vi "1.Main demo.vi"() -> ()   [LabVIEW 2013]
uses:
  UnderAutomation.Fanuc/UnderAutomation.Fanuc.lvlib
  C:/Users/fg/Documents/Fanuc.vi/LabVIEW_2024/UnderAutomation.Fanuc/lib/UnderAutomation.Fanuc.dll
  LabVIEW_2024/UnderAutomation.Fanuc/lib/UnderAutomation.Fanuc.dll
panel:
  out "SNPX connected":bool
  out "FTP connected":bool
  out "Telnet connected":bool
  in  "Tab Control":T1(tab)
  in  "Disconnect":bool
  in  "Test":bool
  in  "Key":string
  in  "Licensee":string
  in  "Use SNPX":bool
  in  "FTP password":string
  in  "FTP user":string
  in  "Use FTP":bool
  in  "Connect":bool
  in  "Telnet password":string
  in  "Use Telnet":bool
  in  "ConnectRoboguide":bool
  in  "RoboguideRobotPath":path caption="Path to \"Robot\" ROBOGUIDE folder that contains services.txt"
  in  "IP":string caption="Robot IP Address"
  out "License state":string
  out "Connect error":string
  in  "Unsimulate all":bool
  in  "Unsimulate":bool
  in  "Simulate":bool
  in  "Set port value":bool
  in  "Variable set value":bool
  in  "Variable new value":string caption="New value"
  in  "Variable get value":bool
  in  "Variable name":string
  out "Telnet warning":string
  out "Current position":T2
  in  "Get current position":bool
  in  "Reset alarms":bool
  in  "Get task info":bool
  in  "Task name":string caption="Task name (program without extension)"
  in  "Abort all programs":bool
  in  "Clear variable":bool
  in  "Clear Program":bool
  in  "Hold":bool
  in  "Continue":bool
  in  "Abort":bool
  in  "Pause":bool
  in  "Program name":string caption="Program name without extension"
  in  "Run":bool
  out "TelnetError":string caption="Error :"
  out "TelnetSucceed":bool caption="Succeeded"
  out "KclCommand":string caption="Last command :"
  out "TaskInfo":T3
  out "Variable value":string
  in  "port":i32(ring) items=["DIN", "DOUT", "RDO", "OPOUT", "TPOUT", "WDI", "WDO", "AIN", "AOUT", "GIN", "GOUT"]
  in  "index":i32
  in  "value":i32
  out "FTP warning":string
  out "PosReg":T4(array[cluster])
  out "StrReg":string[](array[string])
  in  "Tab Control IO state":T5(tab)
  out "UI":cluster{"Id":i32, "Name":string, "Value":bool}[](array[cluster])
  out "UO":cluster{"Id":i32, "Name":string, "Value":bool}[](array[cluster])
  out "SI":cluster{"Id":i32, "Name":string, "Value":bool}[](array[cluster])
  out "SO":cluster{"Id":i32, "Name":string, "Value":bool}[](array[cluster])
  out "DIN":cluster{"Id":i32, "Name":string, "Value":bool}[](array[cluster])
  out "DOUT":cluster{"Id":i32, "Name":string, "Value":bool}[](array[cluster])
  out "RI":cluster{"Id":i32, "Name":string, "Value":bool}[](array[cluster])
  out "RO":cluster{"Id":i32, "Name":string, "Value":bool}[](array[cluster])
  out "FLG":cluster{"Id":i32, "Name":string, "Value":bool}[](array[cluster])
  in  "Tab Control position":enum32{"World", "Joints", "User frames"}(tab)
  out "World Positions":T6(array[cluster])
  out "JointsPosition":dbl[](array[numeric])
  out "UserFramePositions":T7(array[cluster])
  in  "Get current position":bool
  in  "Get IO State":bool
  in  "Port":i32(ring) items=["DIN", "DOUT", "UI", "UO", "SI", "SO", "RI", "RO", "FLG"]
  out "Errors":T8(array[cluster])
  in  "Get all errors":bool
  in  "Get safety status":bool
  out "SafetyStatus":T9
  out "NumReg":dbl[](array[numeric])
  in  "Get numeric registers":bool
  in  "Get string registers":bool
  in  "Get position registers":bool
  out "SNPX warning":string
  in  "Tab Control snpx register":enum32{"Cartesian", "Joints"}(tab)
  in  "Cartesian position 2":T10
  in  "Write cartesian position register":bool
  in  "Joints position":dbl[](array[numeric])
  in  "Write joints position register":bool
  in  "Position register":i32
  in  "Read position register":bool
  out "Value":string
  in  "New value":string
  in  "String register":i32
  in  "Read string register":bool
  in  "Write string register":bool
  in  "Continuous read world position":bool
  out "JointsPosition":dbl[](array[numeric])
  out "Cartesian position":T11
  out "UserTool":i16
  out "error out":errorcluster
  in  "Continuous read user frame position":bool
  in  "userFrame":i32
  out "Cartesian position":T11
  out "UserTool":i16
  out "error out 2":errorcluster
  in  "Numeric register":i32
  in  "New value":sgl
  out "Value":sgl
  in  "Read numeric register":bool
  in  "Write numeric register":bool
  out "UserFrame":i16
  out "UserTool":i16
  in  "stop":bool
  out "Snpx":refnum<k24>
  out "Ftp":refnum<k24>
  out "Telnet":refnum<k24>
  out "robot":refnum<k24>
  # "UnderAutomation"
  # "https://underautomation.com/fanuc"
  # "+"
  # "LabVIEW demo app for remote control and monitoring of your Fanuc robot"
  # "Connect to robot"
  # "2. Ensure you have a trial or lifetime valid license"
  # "1. Set Fanuc robot address"
  # "This is a commercial library, you have a 30-day trial period. But you can use it forever if you buy a perpetual licence for your company (regardless of the number of robot, applications or developers)."
  # "Connect to real robot"
  # "Connect to ROBOGUIDE"
  # "If you have a license :"
  # "3. Select the services you want to connect to"
  # "Telnet"
  # "FTP"
  # "SNPX"
  # "You need option R553 \"HMI Device SNPX\" or R651 FRL"
  # "How to enable Telnet : https://underautomation.com/fanuc/documentation/enable-telnet"
  # "See : https://underautomation.com/fanuc/documentation/snpx"
  # "4. Connect to the robot"
  # "Telnet"
  # "Variables"
  # "Program execution"
  # "Task"
  # "Ports"
  # "Current position"
  # "Alarms"
  # "FTP"
  # "Current Position"
  # "IO State"
  # "Errors"
  # "Registers"
  # "Safety status"
  # "SNPX"
  # "Numeric registers"
  # "String registers"
  # "Read world position"
  # "Read user frame position"
  # "Position registers"
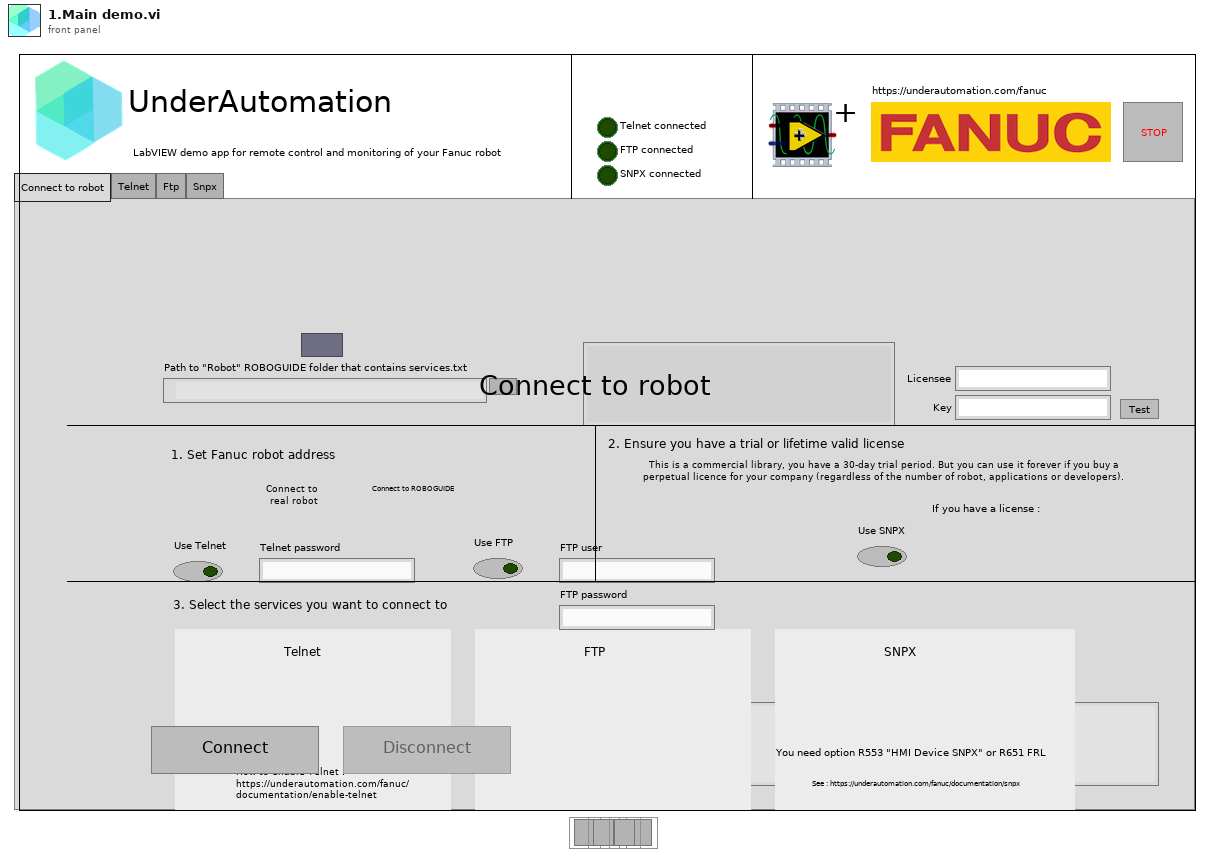
[diagram p1: front panel]
types:
  T1 = enum32{"Connect to robot", "Telnet", "Ftp", "Snpx"}
  T2 = cluster{"X":dbl, "Y":dbl, "Z":dbl, "W":dbl, "P":dbl, "R":dbl}
  T3 = cluster{"CurrentLine":i32, "RoutineName":string, "SystemTask":bool, "TaskName":string, "TaskNumber":i32, "TaskStatus":i32, "TaskStatusStr":string}
  T4 = cluster{"X":dbl, "Y":dbl, "Z":dbl, "W":dbl, "R":dbl, "P":dbl}[][]
  T5 = enum32{"UI", "UO", "SI", "SO", "DIN", "DOUT", "RI", "RO", "FLG"}
  T6 = cluster{"Tool":i32, "Cartesian position":cluster{cluster{"ArmFrontBack":i32, "ArmLeftRight":i32, "ArmUpDown":i32, "TurnAxis1":i32, "TurnAxis2":i32, "TurnAxis3":i32, "WristFlip":i32}, "X":dbl, "Y":dbl, "Z":dbl, "W":dbl, "P":dbl, "R":dbl}}[]
  T7 = cluster{"Frame":i32, "Tool":i32, "Cartesian position":cluster{cluster{"ArmFrontBack":i32, "ArmLeftRight":i32, "ArmUpDown":i32, "TurnAxis1":i32, "TurnAxis2":i32, "TurnAxis3":i32, "WristFlip":i32}, "X":dbl, "Y":dbl, "Z":dbl, "W":dbl, "P":dbl, "R":dbl}}[]
  T8 = cluster{"Id":i32, "IsReset":bool, "Text":string}[]
  T9 = cluster{"BeltBroken":bool, "ExternalEStop":bool, "FenceOpen":bool, "HandBroken":bool, "LowAirAlarm":bool, "NonTeacherEnb":bool, "OverTravel":bool, "SOPEStop":bool, "SVOFFDetect":bool, "TPDeadman":bool, "TPEnable":bool, "TPEStop":bool}
  T10 = cluster{"Configuration":cluster{"ArmFrontBack":i32, "ArmLeftRight":i32, "ArmUpDown":i32, "TurnAxis1":i32, "TurnAxis2":i32, "TurnAxis3":i32, "WristFlip":i32}, "X":dbl, "Y":dbl, "Z":dbl, "W":dbl, "P":dbl, "R":dbl}
  T11 = cluster{"Cartesian position":cluster{cluster{"ArmFrontBack":i32, "ArmLeftRight":i32, "ArmUpDown":i32, "TurnAxis1":i32, "TurnAxis2":i32, "TurnAxis3":i32, "WristFlip":i32}, "X":dbl, "Y":dbl, "Z":dbl, "W":dbl, "P":dbl, "R":dbl}, "Extension":cluster{"E1":dbl, "E2":dbl, "E3":dbl, "T4":i16, "T5":i16, "T6":i16}}
  T12 = enum8{"Enabled", "Disabled", "Disabled and Grayed Out"}
  T13 = cluster{"X":dbl, "Y":dbl, "Z":dbl, "W":dbl, "P":dbl, "R":dbl}[][]
  T14 = cluster{"Id":i32, "Values":dbl[], "UserFramePositions":cluster{"Frame":i32, "Tool":i32, "Cartesian position":cluster{cluster{"ArmFrontBack":i32, "ArmLeftRight":i32, "ArmUpDown":i32, "TurnAxis1":i32, "TurnAxis2":i32, "TurnAxis3":i32, "WristFlip":i32}, "X":dbl, "Y":dbl, "Z":dbl, "W":dbl, "P":dbl, "R":dbl}}[], "World Positions":cluster{"Tool":i32, "Cartesian position":cluster{cluster{"ArmFrontBack":i32, "ArmLeftRight":i32, "ArmUpDown":i32, "TurnAxis1":i32, "TurnAxis2":i32, "TurnAxis3":i32, "WristFlip":i32}, "X":dbl, "Y":dbl, "Z":dbl, "W":dbl, "P":dbl, "R":dbl}}[]}[]
  T15 = cluster{"Id":i32, "Name":string, "Port":i32, "Value":bool, "PortStr":string}[]
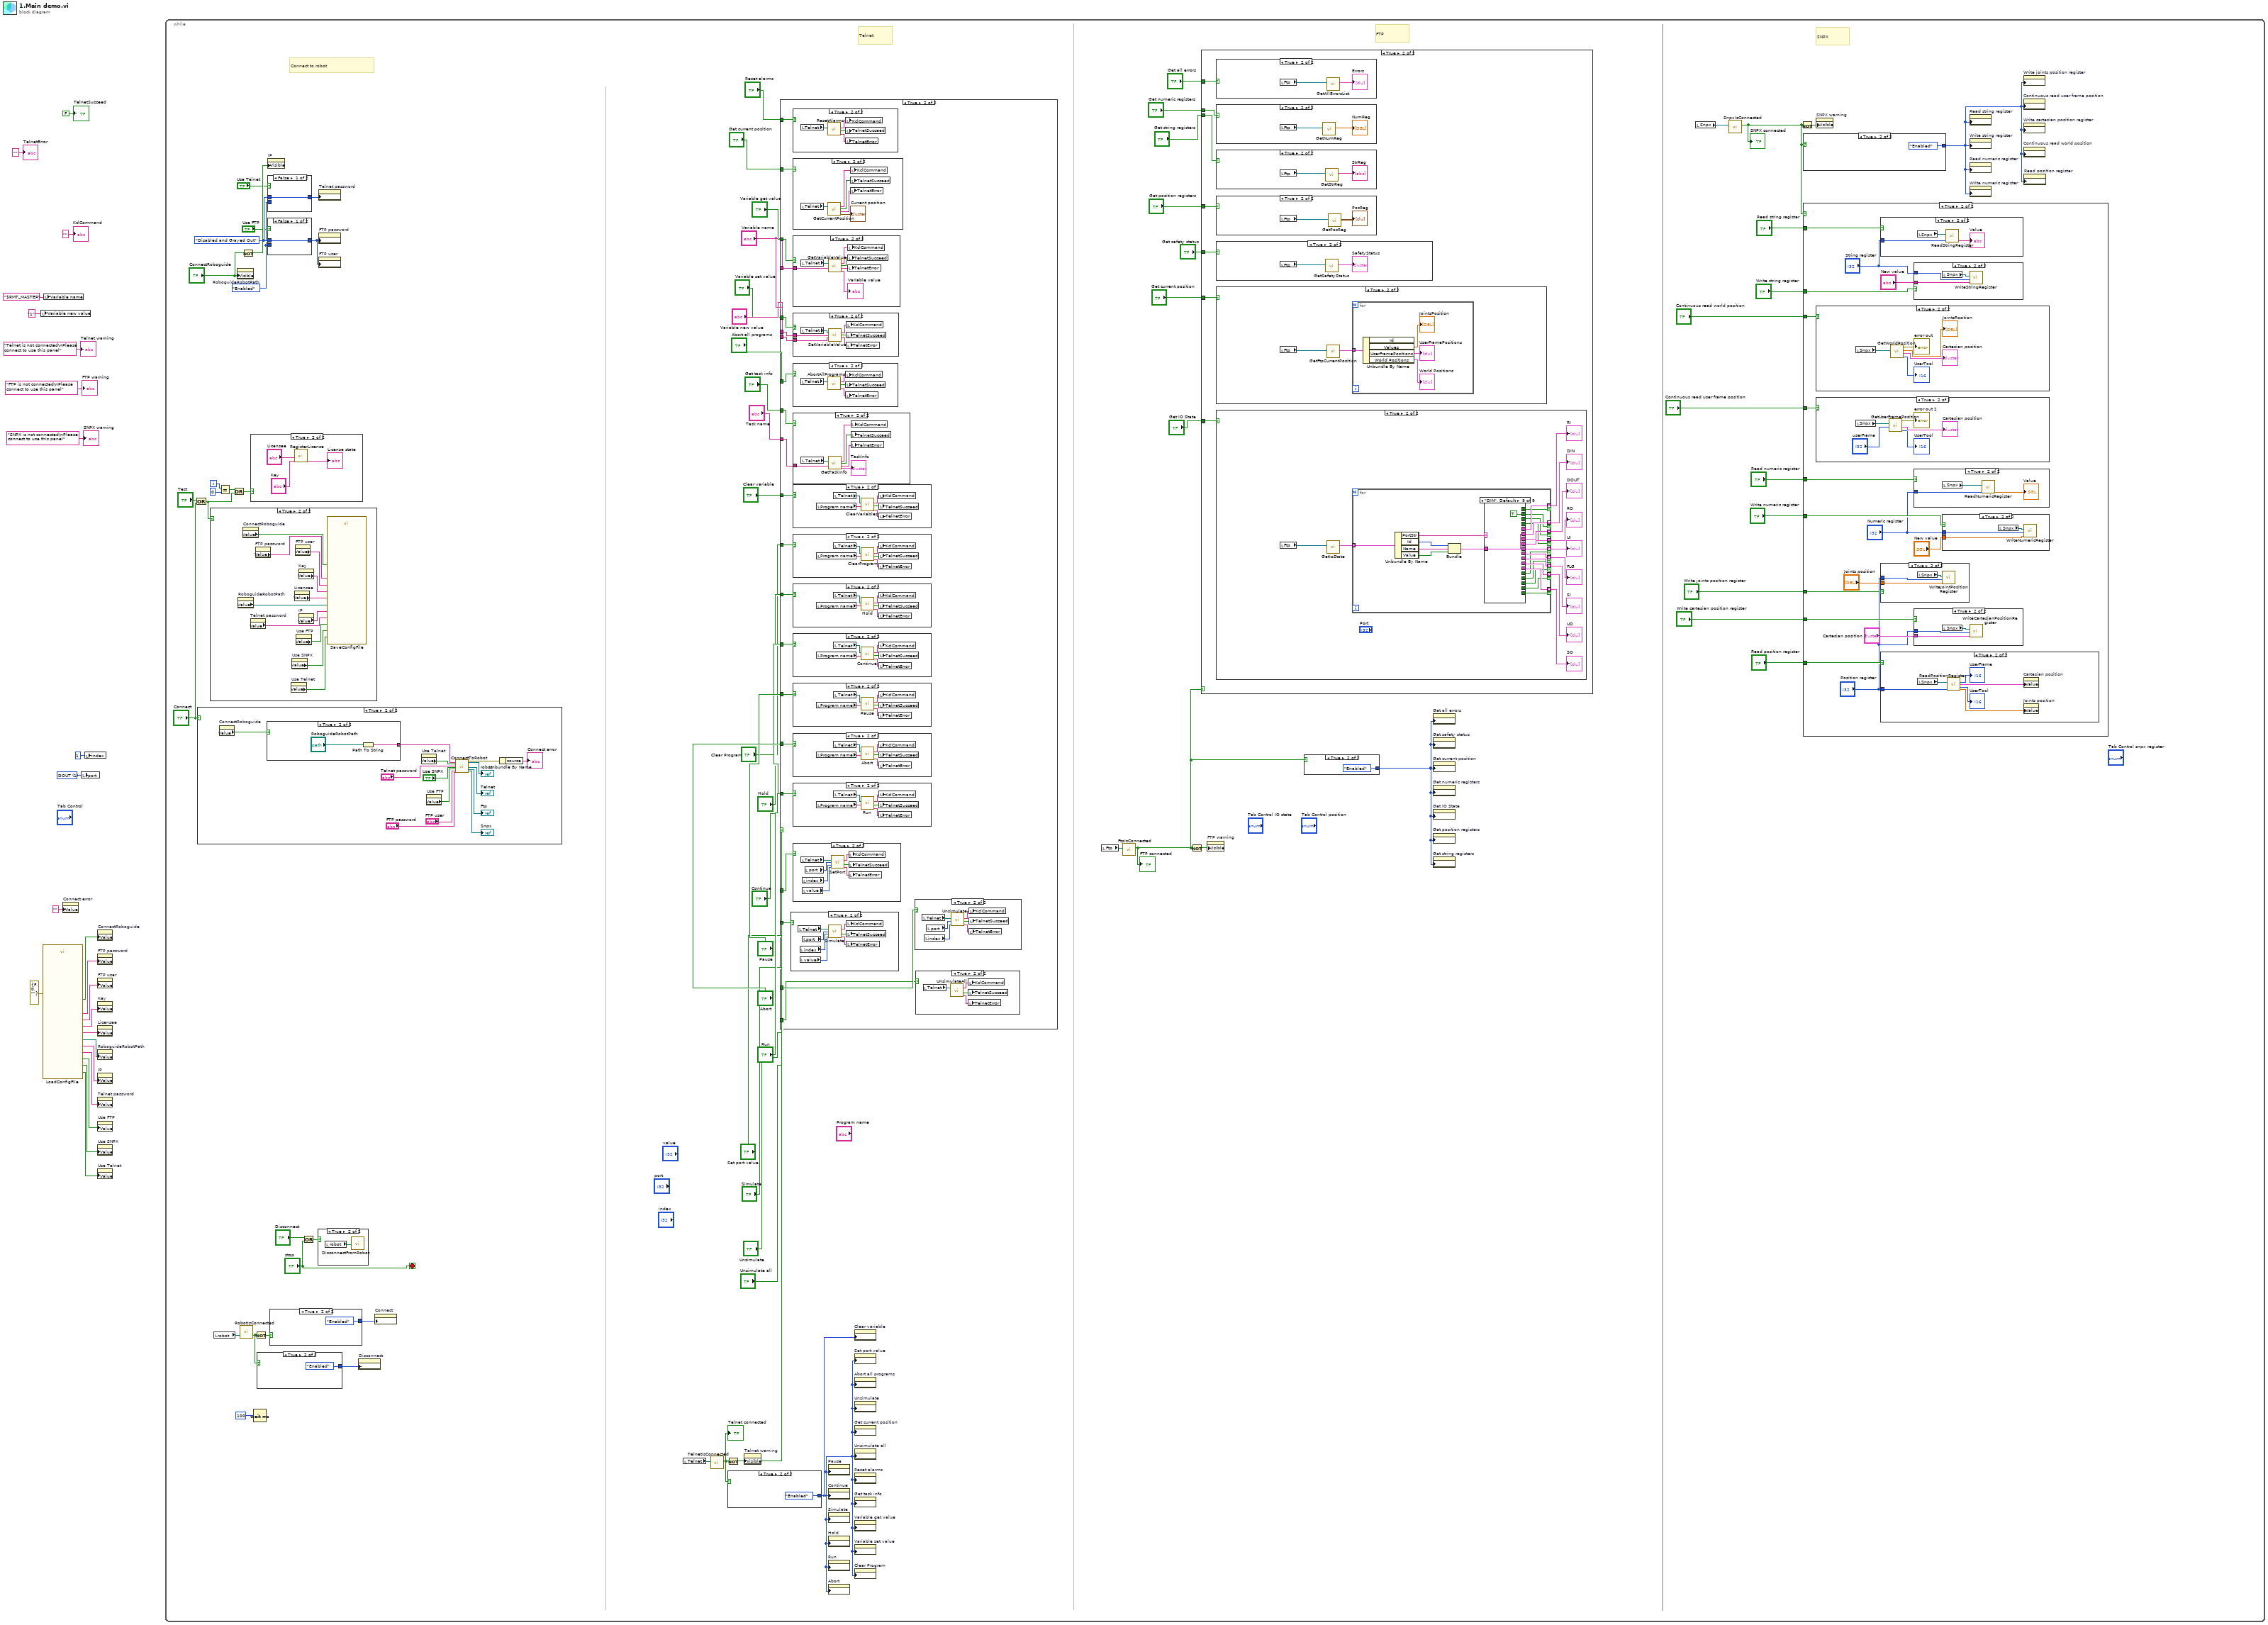
[diagram p0: block diagram]
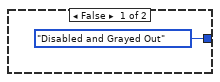
[diagram p2: hidden frame]
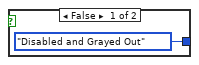
[diagram p13: hidden frame]
diagram:
  w3 = 1 items=["DIN", "DOUT", "RDO", "OPOUT", "TPOUT", "WDI", "WDO", "AIN", "AOUT", "GIN", "GOUT"] ("port")
  n1 = local write "Variable new value"("1" ("Variable new value")) -> ()
  n2 = call "LoadConfigFile.vi"("error in (no error)"=errorcluster {"status"=FALSE, "code"=0, "source"=""}) -> ("FTP password"=w20:string, "Licensee"=w12:string, "FTP user"=w19:string, "Key"=w13:string, "Use FTP"=w16:bool, "IP"=w22:string, "RoboguideRobotPath"=w18:path, "ConnectRoboguide"=w21:bool, "Use Telnet"=w14:bool, "Telnet password"=w17:string, "Use SNPX"=w15:bool)  [unwired: 15 in, 1 out]
  n3 = local write "Variable name"("$RMT_MASTER" ("Variable name")) -> ()
  n4 = property on="Connect error" class="Str"("Value"="" ("Connect error")) -> ()  [unwired: 2 in, 2 out]
  n5 = local write "port"(w3) -> ()
  n6 = local write "index"(1 ("index")) -> ()
  n7 = property on="ConnectRoboguide" class="Bool (strict)"("Value"=w21) -> ()  [unwired: 2 in, 2 out]
  n8 = property on="FTP password" class="Str"("Value"=w20) -> ()  [unwired: 2 in, 2 out]
  n9 = property on="FTP user" class="Str"("Value"=w19) -> ()  [unwired: 2 in, 2 out]
  n10 = property on="Key" class="Str"("Value"=w13) -> ()  [unwired: 2 in, 2 out]
  n11 = property on="Licensee" class="Str"("Value"=w12) -> ()  [unwired: 2 in, 2 out]
  n12 = property on="RoboguideRobotPath" class="Path"("Value"=w18) -> ()  [unwired: 2 in, 2 out]
  n13 = property on="IP" class="Str"("Value"=w22) -> ()  [unwired: 2 in, 2 out]
  n14 = property on="Telnet password" class="Str"("Value"=w17) -> ()  [unwired: 2 in, 2 out]
  n15 = property on="Use FTP" class="Bool (strict)"("Value"=w16) -> ()  [unwired: 2 in, 2 out]
  n16 = property on="Use SNPX" class="Bool (strict)"("Value"=w15) -> ()  [unwired: 2 in, 2 out]
  n17 = property on="Use Telnet" class="Bool (strict)"("Value"=w14) -> ()  [unwired: 2 in, 2 out]
  n18 = while {
    i -> [w90]
    stop <- "stop" stop-if-true
    w82 = T12."Enabled" ("Disabled")
    w83 = T12."Disabled and Grayed Out" ("Disabled")
    # "SNPX"
    # "FTP"
    # "Telnet"
    # "Connect to robot"
    n19 = Or(x="Test", y="Connect") -> (x .or. y?=w87:bool)
    n20 = case shown="True" "Connect" {
      frame False {
      }
      frame True {
        n21 = property on="ConnectRoboguide" class="Bool (strict)"() -> ("Value"=w375:bool)  [unwired: 2 in, 2 out]
        n22 = case shown="True" w375 {
          tunnel: ["IP" w377] -> w374
          frame False {
          }
          frame True {
            n23 = Path To String(path="RoboguideRobotPath") -> (string=w377:string)
          }
        }
        n24 = property on="Use Telnet" class="Bool (strict)"() -> ("Value"=w370:bool)  [unwired: 2 in, 2 out]
        n25 = property on="Use FTP" class="Bool (strict)"() -> ("Value"=w369:bool)  [unwired: 2 in, 2 out]
        n26 = call "ConnectToRobot.vi"("address"=w374, "Telnet enable"=w370, "Telnet KCL password"="Telnet password", "SNPX enable"="Use SNPX", "FTP enable"=w369, "FTP user"="FTP user", "FTP password"="FTP password") -> ("error out"=w368:errorcluster, "robot"=→"robot":refnum<k24>, "Telnet"=→"Telnet":refnum<k24>, "Ftp"=→"Ftp":refnum<k24>, "Snpx"=→"Snpx":refnum<k24>)  [unwired: 16 in]
        n27 = Unbundle By Name(w368) -> ("source"=→"Connect error":string)
      }
    }
    n28 = case shown="True" w87 {
      frame False {
      }
      frame True {
        n29 = property on="RoboguideRobotPath" class="Path"() -> ("Value"=w356:path)  [unwired: 2 in, 2 out]
        n30 = property on="ConnectRoboguide" class="Bool (strict)"() -> ("Value"=w361:bool)  [unwired: 2 in, 2 out]
        n31 = property on="Telnet password" class="Str"() -> ("Value"=w354:string)  [unwired: 2 in, 2 out]
        n32 = property on="FTP password" class="Str"() -> ("Value"=w360:string)  [unwired: 2 in, 2 out]
        n33 = property on="Use Telnet" class="Bool (strict)"() -> ("Value"=w351:bool)  [unwired: 2 in, 2 out]
        n34 = property on="Use SNPX" class="Bool (strict)"() -> ("Value"=w352:bool)  [unwired: 2 in, 2 out]
        n35 = property on="Licensee" class="Str"() -> ("Value"=w357:string)  [unwired: 2 in, 2 out]
        n36 = property on="FTP user" class="Str"() -> ("Value"=w359:string)  [unwired: 2 in, 2 out]
        n37 = property on="Use FTP" class="Bool (strict)"() -> ("Value"=w353:bool)  [unwired: 2 in, 2 out]
        n38 = property on="Key" class="Str"() -> ("Value"=w358:string)  [unwired: 2 in, 2 out]
        n39 = property on="IP" class="Str"() -> ("Value"=w355:string)  [unwired: 2 in, 2 out]
        n40 = call "SaveConfigFile.vi"("IP"=w355, "RoboguideRobotPath"=w356, "ConnectRoboguide"=w361, "Use Telnet"=w351, "Telnet password"=w354, "Use FTP"=w353, "FTP user"=w359, "FTP password"=w360, "Use SNPX"=w352, "Licensee"=w357, "Key"=w358) -> ()  [unwired: 17 in]
      }
    }
    n41 = local read "robot"() -> (w57:refnum<k24>)
    n42 = Equal?(x=w90, y=0) -> (x = y?=w88:bool)
    n43 = Or(x=w88, y=w87) -> (x .or. y?=w86:bool)
    n44 = property on="RoboguideRobotPath" class="Path"("Visible"="ConnectRoboguide") -> ()  [unwired: 2 in, 2 out]
    n45 = call "RobotIsConnected.vi"("robot"=w57) -> ("Connected"=w55:bool)  [unwired: 1 in, 1 out]
    n46 = Not(x="ConnectRoboguide") -> (.not. x?=w94:bool)
    n47 = case shown="True" w86 {
      frame False {
      }
      frame True {
        n48 = call "RegisterLicense.vi"("key"="Key", "licensee"="Licensee") -> ("status"=→"License state":string)  [unwired: 7 in, 2 out]
      }
    }
    n49 = Wait (ms)(milliseconds to wait=u32 100) -> ()  [unwired: 1 out]
    n50 = Not(x=w55) -> (.not. x?=w56:bool)
    n51 = case shown="True" w55 {
      tunnel: [T12."Disabled and Grayed Out" ("Disabled") T12."Enabled" ("Disabled")] -> w54
      frame False {
      }
      frame True {
      }
    }
    n52 = property on="IP" class="Str"("Visible"=w94) -> ()  [unwired: 2 in, 2 out]
    n53 = case shown="False" "Use Telnet" {
      tunnel: w82 -> [_ w347]
      tunnel: [w346 w347] -> w84
      tunnel: w83 -> [w346 _]
      frame False {
      }
      frame True {
      }
    }
    n54 = case shown="False" "Use FTP" {
      tunnel: w82 -> [_ w345]
      tunnel: [w344 w345] -> w80
      tunnel: w83 -> [w344 _]
      frame False {
      }
      frame True {
      }
    }
    n55 = case shown="True" w56 {
      tunnel: [T12."Disabled and Grayed Out" ("Disabled") T12."Enabled" ("Disabled")] -> w53
      frame False {
      }
      frame True {
      }
    }
    n56 = Or(x="Disconnect", y="stop") -> (x .or. y?=w59:bool)
    n57 = case shown="True" w59 {
      frame False {
      }
      frame True {
        n58 = local read "robot"() -> (w230:refnum<k24>)
        n59 = call "DisconnectFromRobot.vi"("robot"=w230) -> ()  [unwired: 26 in, 1 out]
      }
    }
    n60 = property on="Telnet password" class="Str"("DisabledEnum"=w84) -> ()  [unwired: 2 in, 2 out]
    n61 = property on="FTP password" class="Str"("DisabledEnum"=w80) -> ()  [unwired: 2 in, 2 out]
    n62 = property on="FTP user" class="Str"("DisabledEnum"=w80) -> ()  [unwired: 2 in, 2 out]
    n63 = property on="Disconnect" class="Bool"("DisabledEnum"=w54) -> ()  [unwired: 2 in, 2 out]
    n64 = property on="Connect" class="Bool"("DisabledEnum"=w53) -> ()  [unwired: 2 in, 2 out]
    n65 = local read "Telnet"() -> (w79:refnum<k24>)
    n66 = call "TelnetIsConnected.vi"("Telnet"=w79) -> ("Connected"=w77:bool)  [unwired: 9 in, 1 out]
    "Telnet connected" <- w77
    n67 = Not(x=w77) -> (.not. x?=w76:bool)
    n68 = case shown="True" w77 {
      tunnel: [T12."Disabled and Grayed Out" ("Disabled") T12."Enabled" ("Disabled")] -> w48
      frame False {
      }
      frame True {
      }
    }
    n69 = property on="Telnet warning" class="Str"("Visible"=w76) -> ()  [unwired: 2 in, 2 out]
    n70 = case shown="True" w77 {
      tunnel: "Run" -> [_ w253]
      tunnel: "Abort" -> [_ w252]
      tunnel: "Pause" -> [_ w251]
      tunnel: "Continue" -> [_ w250]
      tunnel: "Hold" -> [_ w249]
      tunnel: "Clear variable" -> [_ w248]
      tunnel: "Clear Program" -> [_ w247]
      tunnel: "Abort all programs" -> [_ w246]
      tunnel: "Task name" -> [_ w245]
      tunnel: "Get task info" -> [_ w244]
      tunnel: "Reset alarms" -> [_ w243]
      tunnel: "Get current position" -> [_ w242]
      tunnel: "Variable get value" -> [_ w241]
      tunnel: "Variable name" -> [_ w240]
      tunnel: "Variable name" -> [_ w239]
      tunnel: "Variable new value" -> [_ w238]
      tunnel: "Variable set value" -> [_ w237]
      tunnel: "Set port value" -> [_ w236]
      tunnel: "Simulate" -> [_ w235]
      tunnel: "Unsimulate" -> [_ w234]
      tunnel: "Unsimulate all" -> [_ w233]
      frame False {
      }
      frame True {
        n71 = case shown="True" w235 {
          frame False {
          }
          frame True {
            n72 = local read "Telnet"() -> (w267:refnum<k24>)
            n73 = local read "index"() -> (w264:i32)
            n74 = local read "value"() -> (w266:i32)
            n75 = local read "port"() -> (w265:i32)
            n76 = call "Simulate.vi"("Telnet"=w267, "port"=w265, "index"=w264, "value"=w266) -> ("KclCommand"=w270:string, "Succeed"=w269:bool, "ErrorText"=w268:string)  [unwired: 8 in, 1 out]
            n77 = local write "KclCommand"(w270) -> ()
            n78 = local write "TelnetSucceed"(w269) -> ()
            n79 = local write "TelnetError"(w268) -> ()
          }
        }
        n80 = case shown="True" w243 {
          frame False {
          }
          frame True {
            n81 = local read "Telnet"() -> (w298:refnum<k24>)
            n82 = call "ResetAlarms.vi"("Telnet"=w298) -> ("ErrorText"=w296:string, "Succeed"=w297:bool, "KclCommand"=w295:string)  [unwired: 7 in, 1 out]
            n83 = local write "KclCommand"(w295) -> ()
            n84 = local write "TelnetSucceed"(w297) -> ()
            n85 = local write "TelnetError"(w296) -> ()
          }
        }
        n86 = case shown="True" w242 {
          frame False {
          }
          frame True {
            n87 = local read "Telnet"() -> (w294:refnum<k24>)
            n88 = call "GetCurrentPosition.vi"("Telnet"=w294) -> ("KclCommand"=w292:string, "Succeed"=w291:bool, "ErrorText"=w290:string, "Position"=→"Current position":T2)  [unwired: 10 in, 1 out]
            n89 = local write "KclCommand"(w292) -> ()
            n90 = local write "TelnetSucceed"(w291) -> ()
            n91 = local write "TelnetError"(w290) -> ()
          }
        }
        n92 = case shown="True" w241 {
          tunnel: w240 -> [_ w288]
          frame False {
          }
          frame True {
            n93 = local read "Telnet"() -> (w289:refnum<k24>)
            n94 = call "GetVariableValue.vi"("Telnet"=w289, "name"=w288) -> ("KclCommand"=w284:string, "Succeed"=w285:bool, "ErrorText"=w286:string, "RawValue"=→"Variable value":string)  [unwired: 9 in, 1 out]
            n95 = local write "KclCommand"(w284) -> ()
            n96 = local write "TelnetSucceed"(w285) -> ()
            n97 = local write "TelnetError"(w286) -> ()
          }
        }
        n98 = case shown="True" w237 {
          tunnel: w239 -> [_ w282]
          tunnel: w238 -> [_ w281]
          frame False {
          }
          frame True {
            n99 = local read "Telnet"() -> (w283:refnum<k24>)
            n100 = call "SetVariableValue.vi"("Telnet"=w283, "value"=w281, "name"=w282) -> ("KclCommand"=w280:string, "Succeed"=w279:bool, "ErrorText"=w278:string)  [unwired: 9 in, 1 out]
            n101 = local write "KclCommand"(w280) -> ()
            n102 = local write "TelnetSucceed"(w279) -> ()
            n103 = local write "TelnetError"(w278) -> ()
          }
        }
        n104 = case shown="True" w246 {
          frame False {
          }
          frame True {
            n105 = local read "Telnet"() -> (w305:refnum<k24>)
            n106 = call "AbortAllPrograms.vi"("Telnet"=w305) -> ("ErrorText"=w306:string, "Succeed"=w307:bool, "KclCommand"=w308:string)  [unwired: 7 in, 1 out]
            n107 = local write "KclCommand"(w308) -> ()
            n108 = local write "TelnetSucceed"(w307) -> ()
            n109 = local write "TelnetError"(w306) -> ()
          }
        }
        n110 = case shown="True" w244 {
          tunnel: w245 -> [_ w303]
          frame False {
          }
          frame True {
            n111 = local read "Telnet"() -> (w304:refnum<k24>)
            n112 = call "GetTaskInfo.vi"("Telnet"=w304, "task"=w303) -> ("KclCommand"=w301:string, "Succeed"=w300:bool, "ErrorText"=w299:string, "TaskInfo"=→"TaskInfo":T3)  [unwired: 9 in, 1 out]
            n113 = local write "KclCommand"(w301) -> ()
            n114 = local write "TelnetSucceed"(w300) -> ()
            n115 = local write "TelnetError"(w299) -> ()
          }
        }
        n116 = case shown="True" w248 {
          frame False {
          }
          frame True {
            n117 = local read "Program name"() -> (w309:string)
            n118 = local read "Telnet"() -> (w310:refnum<k24>)
            n119 = call "ClearVariables.vi"("program"=w309, "Telnet"=w310) -> ("ErrorText"=w311:string, "Succeed"=w312:bool, "KclCommand"=w313:string)  [unwired: 6 in, 1 out]
            n120 = local write "KclCommand"(w313) -> ()
            n121 = local write "TelnetSucceed"(w312) -> ()
            n122 = local write "TelnetError"(w311) -> ()
          }
        }
        n123 = case shown="True" w247 {
          frame False {
          }
          frame True {
            n124 = local read "Program name"() -> (w314:string)
            n125 = local read "Telnet"() -> (w315:refnum<k24>)
            n126 = call "ClearProgram.vi"("program"=w314, "Telnet"=w315) -> ("ErrorText"=w316:string, "Succeed"=w317:bool, "KclCommand"=w318:string)  [unwired: 6 in, 1 out]
            n127 = local write "KclCommand"(w318) -> ()
            n128 = local write "TelnetSucceed"(w317) -> ()
            n129 = local write "TelnetError"(w316) -> ()
          }
        }
        n130 = case shown="True" w249 {
          frame False {
          }
          frame True {
            n131 = local read "Program name"() -> (w319:string)
            n132 = local read "Telnet"() -> (w320:refnum<k24>)
            n133 = call "Hold.vi"("program"=w319, "Telnet"=w320) -> ("ErrorText"=w321:string, "Succeed"=w322:bool, "KclCommand"=w323:string)  [unwired: 6 in, 1 out]
            n134 = local write "KclCommand"(w323) -> ()
            n135 = local write "TelnetSucceed"(w322) -> ()
            n136 = local write "TelnetError"(w321) -> ()
          }
        }
        n137 = case shown="True" w250 {
          frame False {
          }
          frame True {
            n138 = local read "Program name"() -> (w324:string)
            n139 = local read "Telnet"() -> (w325:refnum<k24>)
            n140 = call "Continue.vi"("program"=w324, "Telnet"=w325) -> ("ErrorText"=w326:string, "Succeed"=w327:bool, "KclCommand"=w328:string)  [unwired: 6 in, 1 out]
            n141 = local write "KclCommand"(w328) -> ()
            n142 = local write "TelnetSucceed"(w327) -> ()
            n143 = local write "TelnetError"(w326) -> ()
          }
        }
        n144 = case shown="True" w251 {
          frame False {
          }
          frame True {
            n145 = local read "Program name"() -> (w329:string)
            n146 = local read "Telnet"() -> (w330:refnum<k24>)
            n147 = call "Pause.vi"("program"=w329, "Telnet"=w330) -> ("ErrorText"=w331:string, "Succeed"=w332:bool, "KclCommand"=w333:string)  [unwired: 6 in, 1 out]
            n148 = local write "KclCommand"(w333) -> ()
            n149 = local write "TelnetSucceed"(w332) -> ()
            n150 = local write "TelnetError"(w331) -> ()
          }
        }
        n151 = case shown="True" w252 {
          frame False {
          }
          frame True {
            n152 = local read "Program name"() -> (w334:string)
            n153 = local read "Telnet"() -> (w335:refnum<k24>)
            n154 = call "Abort.vi"("program"=w334, "Telnet"=w335) -> ("ErrorText"=w336:string, "Succeed"=w337:bool, "KclCommand"=w338:string)  [unwired: 6 in, 1 out]
            n155 = local write "KclCommand"(w338) -> ()
            n156 = local write "TelnetSucceed"(w337) -> ()
            n157 = local write "TelnetError"(w336) -> ()
          }
        }
        n158 = case shown="True" w253 {
          frame False {
          }
          frame True {
            n159 = local read "Program name"() -> (w339:string)
            n160 = local read "Telnet"() -> (w340:refnum<k24>)
            n161 = call "Run.vi"("program"=w339, "Telnet"=w340) -> ("ErrorText"=w341:string, "Succeed"=w342:bool, "KclCommand"=w343:string)  [unwired: 6 in, 1 out]
            n162 = local write "KclCommand"(w343) -> ()
            n163 = local write "TelnetSucceed"(w342) -> ()
            n164 = local write "TelnetError"(w341) -> ()
          }
        }
        n165 = case shown="True" w236 {
          frame False {
          }
          frame True {
            n166 = local read "Telnet"() -> (w274:refnum<k24>)
            n167 = local read "index"() -> (w271:i32)
            n168 = local read "value"() -> (w273:i32)
            n169 = local read "port"() -> (w272:i32)
            n170 = call "SetPort.vi"("Telnet"=w274, "port"=w272, "index"=w271, "value"=w273) -> ("KclCommand"=w277:string, "Succeed"=w276:bool, "ErrorText"=w275:string)  [unwired: 8 in, 1 out]
            n171 = local write "KclCommand"(w277) -> ()
            n172 = local write "TelnetSucceed"(w276) -> ()
            n173 = local write "TelnetError"(w275) -> ()
          }
        }
        n174 = case shown="True" w234 {
          frame False {
          }
          frame True {
            n175 = local read "Telnet"() -> (w260:refnum<k24>)
            n176 = local read "index"() -> (w258:i32)
            n177 = local read "port"() -> (w259:i32)
            n178 = call "Unsimulate.vi"("index"=w258, "port"=w259, "Telnet"=w260) -> ("ErrorText"=w261:string, "Succeed"=w262:bool, "KclCommand"=w263:string)  [unwired: 5 in, 1 out]
            n179 = local write "KclCommand"(w263) -> ()
            n180 = local write "TelnetSucceed"(w262) -> ()
            n181 = local write "TelnetError"(w261) -> ()
          }
        }
        n182 = case shown="True" w233 {
          frame False {
          }
          frame True {
            n183 = local read "Telnet"() -> (w254:refnum<k24>)
            n184 = call "UnsimulateAll.vi"("Telnet"=w254) -> ("KclCommand"=w257:string, "Succeed"=w256:bool, "ErrorText"=w255:string)  [unwired: 11 in, 1 out]
            n185 = local write "KclCommand"(w257) -> ()
            n186 = local write "TelnetSucceed"(w256) -> ()
            n187 = local write "TelnetError"(w255) -> ()
          }
        }
      }
    }
    n188 = property on="Pause" class="Bool"("DisabledEnum"=w48) -> ()  [unwired: 2 in, 2 out]
    n189 = property on="Continue" class="Bool"("DisabledEnum"=w48) -> ()  [unwired: 2 in, 2 out]
    n190 = property on="Simulate" class="Bool"("DisabledEnum"=w48) -> ()  [unwired: 2 in, 2 out]
    n191 = property on="Hold" class="Bool"("DisabledEnum"=w48) -> ()  [unwired: 2 in, 2 out]
    n192 = property on="Run" class="Bool"("DisabledEnum"=w48) -> ()  [unwired: 2 in, 2 out]
    n193 = property on="Abort" class="Bool"("DisabledEnum"=w48) -> ()  [unwired: 2 in, 2 out]
    n194 = property on="Clear variable" class="Bool"("DisabledEnum"=w48) -> ()  [unwired: 2 in, 2 out]
    n195 = property on="Set port value" class="Bool"("DisabledEnum"=w48) -> ()  [unwired: 2 in, 2 out]
    n196 = property on="Abort all programs" class="Bool"("DisabledEnum"=w48) -> ()  [unwired: 2 in, 2 out]
    n197 = property on="Unsimulate" class="Bool"("DisabledEnum"=w48) -> ()  [unwired: 2 in, 2 out]
    n198 = property on="Get current position" class="Bool"("DisabledEnum"=w48) -> ()  [unwired: 2 in, 2 out]
    n199 = property on="Unsimulate all" class="Bool"("DisabledEnum"=w48) -> ()  [unwired: 2 in, 2 out]
    n200 = property on="Reset alarms" class="Bool"("DisabledEnum"=w48) -> ()  [unwired: 2 in, 2 out]
    n201 = property on="Get task info" class="Bool"("DisabledEnum"=w48) -> ()  [unwired: 2 in, 2 out]
    n202 = property on="Variable get value" class="Bool"("DisabledEnum"=w48) -> ()  [unwired: 2 in, 2 out]
    n203 = property on="Variable set value" class="Bool"("DisabledEnum"=w48) -> ()  [unwired: 2 in, 2 out]
    n204 = property on="Clear Program" class="Bool"("DisabledEnum"=w48) -> ()  [unwired: 2 in, 2 out]
    n205 = local read "Ftp"() -> (w47:refnum<k24>)
    n206 = call "FtpIsConnected.vi"("Ftp"=w47) -> ("Connected"=w38:bool)  [unwired: 9 in, 1 out]
    "FTP connected" <- w38
    n207 = Not(x=w38) -> (.not. x?=w39:bool)
    n208 = case shown="True" w38 {
      tunnel: "Get current position" -> [_ w156]
      tunnel: "Get IO State" -> [_ w155]
      tunnel: "Get all errors" -> [_ w154]
      tunnel: "Get safety status" -> [_ w153]
      tunnel: "Get numeric registers" -> [_ w152]
      tunnel: "Get string registers" -> [_ w151]
      tunnel: "Get position registers" -> [_ w150]
      frame False {
      }
      frame True {
        n209 = case shown="True" w154 {
          frame False {
          }
          frame True {
            n210 = local read "Ftp"() -> (w166:refnum<k24>)
            n211 = call "GetAllErrorsList.vi"("Ftp"=w166) -> ("Errors"=→"Errors":T8)  [unwired: 9 in, 1 out]
          }
        }
        n212 = case shown="True" w152 {
          frame False {
          }
          frame True {
            n213 = local read "Ftp"() -> (w162:refnum<k24>)
            n214 = call "GetNumReg.vi"("Ftp"=w162) -> ("NumReg"=→"NumReg":dbl[])  [unwired: 9 in, 1 out]
          }
        }
        n215 = case shown="True" w151 {
          frame False {
          }
          frame True {
            n216 = local read "Ftp"() -> (w160:refnum<k24>)
            n217 = call "GetStrReg.vi"("Ftp"=w160) -> ("StrReg"=→"StrReg":string[])  [unwired: 9 in, 1 out]
          }
        }
        n218 = case shown="True" w150 {
          frame False {
          }
          frame True {
            n219 = local read "Ftp"() -> (w158:refnum<k24>)
            n220 = call "GetPosReg.vi"("Ftp"=w158) -> ("PosReg"=→"PosReg":T13)  [unwired: 9 in, 1 out]
          }
        }
        n221 = case shown="True" w153 {
          frame False {
          }
          frame True {
            n222 = local read "Ftp"() -> (w164:refnum<k24>)
            n223 = call "GetSafetyStatus.vi"("Ftp"=w164) -> ("SafetyStatus"=→"SafetyStatus":T9)  [unwired: 9 in, 1 out]
          }
        }
        n224 = case shown="True" w156 {
          frame False {
          }
          frame True {
            n225 = local read "Ftp"() -> (w221:refnum<k24>)
            n226 = call "GetFtpCurrentPosition.vi"("Ftp"=w221) -> ("Current position"=w220:T14)  [unwired: 9 in, 1 out]
            n227 = for {
              tunnel: w220 -> [w224] mode=indexing
              n228 = Unbundle By Name(w224) -> ("Values"=→"JointsPosition":dbl[], "UserFramePositions"=→"UserFramePositions":T7, "World Positions"=→"World Positions":T6)  [unwired: 1 out]
            }
          }
        }
        n229 = case shown="True" w155 {
          frame False {
          }
          frame True {
            n230 = local read "Ftp"() -> (w177:refnum<k24>)
            n231 = call "GetIoState.vi"("Ftp"=w177) -> ("IO States"=w176:T15)  [unwired: 9 in, 1 out]
            n232 = for {
              tunnel: w176 -> [w201] mode=indexing
              tunnel: [w197] -> w175 mode=indexing if=w181
              tunnel: [w195] -> w174 mode=indexing if=w182
              tunnel: [w187] -> w167 mode=indexing if=w180
              tunnel: [w194] -> w173 mode=indexing if=w179
              tunnel: [w193] -> w172 mode=indexing if=w178
              tunnel: [w192] -> w171 mode=indexing if=w186
              tunnel: [w191] -> w170 mode=indexing if=w185
              tunnel: [w190] -> w169 mode=indexing if=w184
              tunnel: [w188] -> w168 mode=indexing if=w183
              n233 = Unbundle By Name(w201) -> ("PortStr"=w189:string, "Id"=w200:i32, "Name"=w199:string, "Value"=w198:bool)
              n234 = Bundle("Id"=w200, "Name"=w199, "Value"=w198) -> (w196:cluster{"Id":i32, "Name":string, "Value":bool})  [unwired: 1 in]
              n235 = case shown="\"DIN\", Default" w189 {
                tunnel: [_ _ _ _ _ _ _ w217 _] -> w197
                tunnel: w196 -> [w203 w205 w207 w209 w211 w213 w215 w217 w219]
                tunnel: [_ _ _ _ _ _ w215 _ _] -> w195
                tunnel: [_ _ _ _ _ _ _ _ w219] -> w187
                tunnel: [w203 _ _ _ _ _ _ _ _] -> w194
                tunnel: [_ w205 _ _ _ _ _ _ _] -> w193
                tunnel: [_ _ w207 _ _ _ _ _ _] -> w192
                tunnel: [_ _ _ w209 _ _ _ _ _] -> w191
                tunnel: [_ _ _ _ w211 _ _ _ _] -> w190
                tunnel: [_ _ _ _ _ w213 _ _ _] -> w188
                tunnel: [_ _ TRUE _ _ _ _ _ _] -> w186
                tunnel: [_ _ _ TRUE _ _ _ _ _] -> w185
                tunnel: [_ _ _ _ TRUE _ _ _ _] -> w184
                tunnel: [_ _ _ _ _ TRUE _ _ _] -> w183
                tunnel: [_ _ _ _ _ _ TRUE _ _] -> w182
                tunnel: [_ _ _ _ _ _ _ TRUE _] -> w181
                tunnel: [_ _ _ _ _ _ _ _ TRUE] -> w180
                tunnel: [TRUE _ _ _ _ _ _ _ _] -> w179
                tunnel: [_ TRUE _ _ _ _ _ _ _] -> w178
                frame "DOUT" {
                }
                frame "UI" {
                }
                frame "UO" {
                }
                frame "SI" {
                }
                frame "SO" {
                }
                frame "RI" {
                }
                frame "RO" {
                }
                frame "FLG" {
                }
                frame "DIN", Default {
                }
              }
            }
            "FLG" <- w175
            "RO" <- w174
            "DIN" <- w167
            "DOUT" <- w173
            "UI" <- w172
            "UO" <- w171
            "SI" <- w170
            "SO" <- w169
            "RI" <- w168
          }
        }
      }
    }
    n236 = property on="FTP warning" class="Str"("Visible"=w39) -> ()  [unwired: 2 in, 2 out]
    n237 = case shown="True" w38 {
      tunnel: [T12."Disabled and Grayed Out" ("Disabled") T12."Enabled" ("Disabled")] -> w37
      frame False {
      }
      frame True {
      }
    }
    n238 = property on="Get all errors" class="Bool"("DisabledEnum"=w37) -> ()  [unwired: 2 in, 2 out]
    n239 = property on="Get safety status" class="Bool"("DisabledEnum"=w37) -> ()  [unwired: 2 in, 2 out]
    n240 = property on="Get current position" class="Bool"("DisabledEnum"=w37) -> ()  [unwired: 2 in, 2 out]
    n241 = property on="Get numeric registers" class="Bool"("DisabledEnum"=w37) -> ()  [unwired: 2 in, 2 out]
    n242 = property on="Get IO State" class="Bool"("DisabledEnum"=w37) -> ()  [unwired: 2 in, 2 out]
    n243 = property on="Get position registers" class="Bool"("DisabledEnum"=w37) -> ()  [unwired: 2 in, 2 out]
    n244 = property on="Get string registers" class="Bool"("DisabledEnum"=w37) -> ()  [unwired: 2 in, 2 out]
    n245 = local read "Snpx"() -> (w35:refnum<k24>)
    n246 = call "SnpxIsConnected.vi"("Snpx"=w35) -> ("Connected"=w25:bool)  [unwired: 9 in, 1 out]
    "SNPX connected" <- w25
    n247 = Not(x=w25) -> (.not. x?=w36:bool)
    n248 = case shown="True" w25 {
      tunnel: [T12."Disabled and Grayed Out" ("Disabled") T12."Enabled" ("Disabled")] -> w24
      frame False {
      }
      frame True {
      }
    }
    n249 = case shown="True" w25 {
      tunnel: "Continuous read world position" -> [_ w113]
      tunnel: "Continuous read user frame position" -> [_ w112]
      tunnel: "Read numeric register" -> [_ w111]
      tunnel: "Write numeric register" -> [_ w110]
      tunnel: "Read string register" -> [_ w105]
      tunnel: "Write string register" -> [_ w104]
      tunnel: "Read position register" -> [_ w103]
      tunnel: "Write cartesian position register" -> [_ w102]
      tunnel: "Write joints position register" -> [_ w98]
      frame False {
      }
      frame True {
        n250 = case shown="True" w113 {
          frame False {
          }
          frame True {
            n251 = local read "Snpx"() -> (w143:refnum<k24>)
            n252 = call "GetWorldPosition.vi"("Snpx"=w143) -> ("UserTool"=→"UserTool":i16, "Cartesian position"=→"Cartesian position":T11, "JointsPosition"=→"JointsPosition":dbl[], "error out"=→"error out":errorcluster)  [unwired: 7 in]
          }
        }
        n253 = case shown="True" w112 {
          frame False {
          }
          frame True {
            n254 = local read "Snpx"() -> (w139:refnum<k24>)
            n255 = call "GetUserFramePosition.vi"("userFrame"="userFrame", "Snpx"=w139) -> ("UserTool"=→"UserTool":i16, "Cartesian position"=→"Cartesian position":T11, "error out"=→"error out 2":errorcluster)  [unwired: 6 in, 1 out]
          }
        }
        n256 = case shown="True" w105 {
          tunnel: "String register" -> [_ w130]
          frame False {
          }
          frame True {
            n257 = local read "Snpx"() -> (w131:refnum<k24>)
            n258 = call "ReadStringRegister.vi"("index"=w130, "Snpx"=w131) -> ("Value"=→"Value":string)  [unwired: 8 in, 1 out]
          }
        }
        n259 = case shown="True" w98 {
          tunnel: "Position register" -> [_ w115]
          tunnel: "Joints position" -> [_ w114]
          frame False {
          }
          frame True {
            n260 = local read "Snpx"() -> (w116:refnum<k24>)
            n261 = call "WriteJointPositionRegister.vi"("Value"=w114, "index"=w115, "Snpx"=w116) -> ()  [unwired: 8 in, 1 out]
          }
        }
        n262 = case shown="True" w103 {
          tunnel: "Position register" -> [_ w124]
          frame False {
          }
          frame True {
            n263 = local read "Snpx"() -> (w125:refnum<k24>)
            n264 = call "ReadPositionRegister.vi"("Snpx"=w125, "index"=w124) -> ("UserFrame"=→"UserFrame":i16, "Cartesian position"=w123:T10, "UserTool"=→"UserTool":i16, "Joint position"=w120:dbl[])  [unwired: 9 in, 1 out]
            n265 = property on="Cartesian position" class="Clust (strict)"("Value"=w123) -> ()  [unwired: 2 in, 2 out]
            n266 = property on="Joints position" class="Arr (strict)"("Value"=w120) -> ()  [unwired: 2 in, 2 out]
          }
        }
        n267 = case shown="True" w104 {
          tunnel: "String register" -> [_ w127]
          tunnel: "New value" -> [_ w126]
          frame False {
          }
          frame True {
            n268 = local read "Snpx"() -> (w128:refnum<k24>)
            n269 = call "WriteStringRegister.vi"("value"=w126, "index"=w127, "Snpx"=w128) -> ()  [unwired: 8 in, 1 out]
          }
        }
        n270 = case shown="True" w111 {
          tunnel: "Numeric register" -> [_ w136]
          frame False {
          }
          frame True {
            n271 = local read "Snpx"() -> (w137:refnum<k24>)
            n272 = call "ReadNumericRegister.vi"("index"=w136, "Snpx"=w137) -> ("Value"=→"Value":sgl)  [unwired: 8 in, 1 out]
          }
        }
        n273 = case shown="True" w102 {
          tunnel: "Cartesian position 2" -> [_ w118]
          tunnel: "Position register" -> [_ w117]
          frame False {
          }
          frame True {
            n274 = local read "Snpx"() -> (w119:refnum<k24>)
            n275 = call "WriteCartesianPositionRegister.vi"("Cartesian position"=w118, "index"=w117, "Snpx"=w119) -> ()  [unwired: 8 in, 1 out]
          }
        }
        n276 = case shown="True" w110 {
          tunnel: "New value" -> [_ w133]
          tunnel: "Numeric register" -> [_ w132]
          frame False {
          }
          frame True {
            n277 = local read "Snpx"() -> (w134:refnum<k24>)
            n278 = call "WriteNumericRegister.vi"("Value"=w133, "index"=w132, "Snpx"=w134) -> ()  [unwired: 8 in, 1 out]
          }
        }
      }
    }
    n279 = property on="SNPX warning" class="Str"("Visible"=w36) -> ()  [unwired: 2 in, 2 out]
    n280 = property on="Read string register" class="Bool"("DisabledEnum"=w24) -> ()  [unwired: 2 in, 2 out]
    n281 = property on="Write string register" class="Bool"("DisabledEnum"=w24) -> ()  [unwired: 2 in, 2 out]
    n282 = property on="Read numeric register" class="Bool"("DisabledEnum"=w24) -> ()  [unwired: 2 in, 2 out]
    n283 = property on="Write numeric register" class="Bool"("DisabledEnum"=w24) -> ()  [unwired: 2 in, 2 out]
    n284 = property on="Write joints position register" class="Bool"("DisabledEnum"=w24) -> ()  [unwired: 2 in, 2 out]
    n285 = property on="Continuous read user frame position" class="Bool (strict)"("DisabledEnum"=w24) -> ()  [unwired: 2 in, 2 out]
    n286 = property on="Write cartesian position register" class="Bool"("DisabledEnum"=w24) -> ()  [unwired: 2 in, 2 out]
    n287 = property on="Continuous read world position" class="Bool (strict)"("DisabledEnum"=w24) -> ()  [unwired: 2 in, 2 out]
    n288 = property on="Read position register" class="Bool"("DisabledEnum"=w24) -> ()  [unwired: 2 in, 2 out]
  }
  "TelnetError" <- "" ("ErrorText")
  "TelnetSucceed" <- FALSE ("Succeed")
  "KclCommand" <- "" ("KclCommand")
  "Telnet warning" <- "Telnet is not connected\nPlease connect to use this panel" ("Telnet warning")
  "FTP warning" <- "FTP is not connected\nPlease connect to use this panel" ("FTP warning")
  "SNPX warning" <- "SNPX is not connected\nPlease connect to use this panel" ("FTP warning")
